vi "Write Message Stream.vi"(8 "error in (no error)":errorcluster, 10 "Message Stream.lvclass":refnum<class "Message Stream.lvclass">, 11 "Host MSS Test Actor in":refnum<class "Host MSS Test Actor.lvclass">) -> (0 "error out":errorcluster, 3 "Host MSS Test Actor out":refnum<class "Host MSS Test Actor.lvclass">)   [LabVIEW 2023, in "Host MSS Test Actor.lvlib" / "Host MSS Test Actor.lvclass"]
uses:
  Host MSS Test Actor.lvclass
  <vilib>/ni/Actors/Network Endpoint Actors/Abstract Classes/Message Stream/Message Stream.lvclass
  Host MSS Test Actor.lvclass/Host MSS Test Actor.ctl
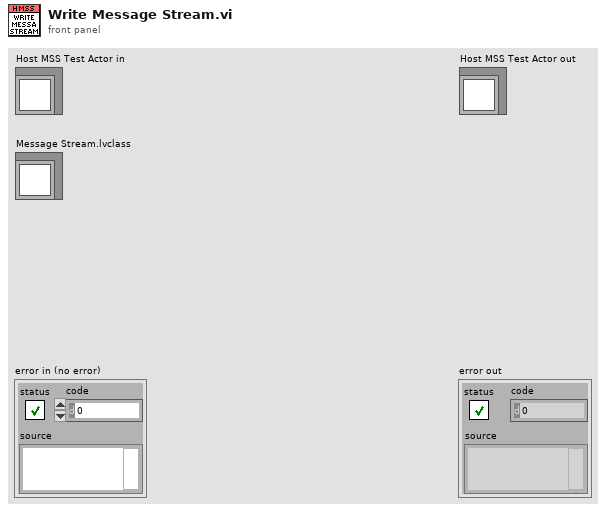
[diagram p1: front panel]
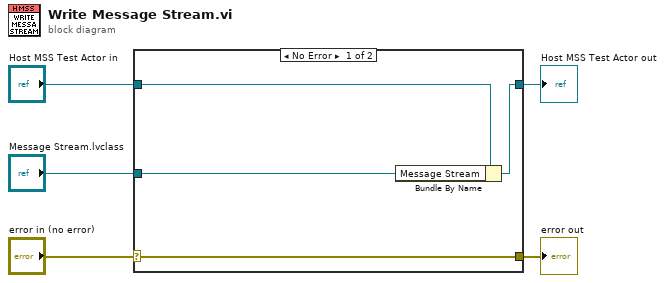
[diagram p0: block diagram]
diagram:
  n1 = case shown="No Error" "error in (no error)" {
    selector: "error in (no error)" -> [w9 w10]
    tunnel: [w9 w10] -> w4
    tunnel: [w7 w11] -> w2
    tunnel: "Host MSS Test Actor in" -> [w8 w11]
    tunnel: "Message Stream.lvclass" -> [w6 _]
    frame No Error {
      n2 = Bundle By Name(cluster=w8, "Message Stream"=w6) -> (w7:refnum<class "Host MSS Test Actor.lvclass">)
    }
    frame Error {
    }
  }
  "error out" <- w4
  "Host MSS Test Actor out" <- w2
